vi "MixAndDownsample_5761_stage1.vi"(4 "cosine":fxp<+/-,16,0>, 6 "sine":fxp<+/-,16,0>, 11 "Analog in":i16) -> (0 "data valid":bool, 1 "Q out":fxp<+/-,16,14>, 2 "I out":fxp<+/-,16,14>)   [LabVIEW 2018]
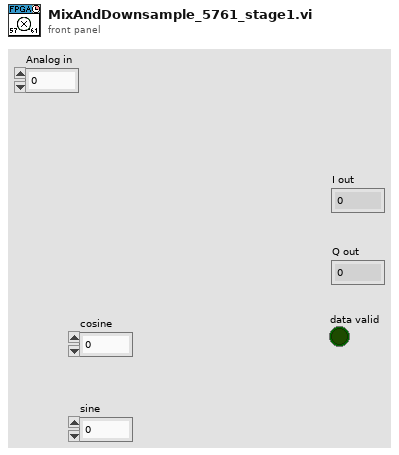
[diagram p1: front panel]
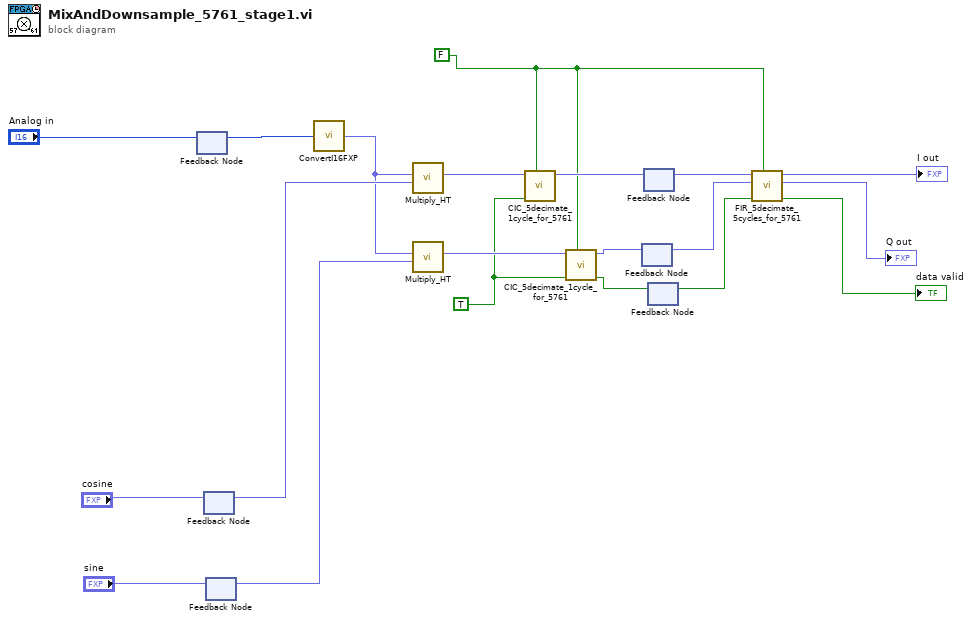
[diagram p0: block diagram]
diagram:
  w4 = FALSE ("reset")
  w11 = TRUE ("valid in")
  n1 = feedback #1() -> (w16:i16)  [unwired: 1 in]
  n2 = feedback-in #1("Analog in") -> ()
  n3 = feedback #2() -> (w17:fxp<+/-,16,0>)  [unwired: 1 in]
  n4 = feedback-in #2("cosine") -> ()
  n5 = feedback #3() -> (w13:fxp<+/-,16,0>)  [unwired: 1 in]
  n6 = feedback-in #3("sine") -> ()
  n7 = call "ConvertI16FXP.vi"("I16"=w16) -> ("y"=w14:fxp<+/-,16,16>)
  n8 = call "Multiply_HT.vi"("DDS sample"=w17, "Signal sample"=w14) -> ("Output"=w15:fxp<+/-,16,14>)  [unwired: 8 in, 1 out]
  n9 = call "Multiply_HT.vi"("DDS sample"=w13, "Signal sample"=w14) -> ("Output"=w12:fxp<+/-,16,14>)  [unwired: 8 in, 1 out]
  n10 = call "CIC_5decimate_1cycle_for_5761.vi"("reset"=w4, "valid in"=w11, "Data in"=w15) -> ("Data out"=w10:fxp<+/-,16,14>)  [unwired: 7 in, 1 out]
  n11 = call "CIC_5decimate_1cycle_for_5761.vi"("reset"=w4, "valid in"=w11, "Data in"=w12) -> ("valid out"=w6:bool, "Data out"=w8:fxp<+/-,16,14>)  [unwired: 7 in]
  n12 = feedback #4() -> (w7:fxp<+/-,16,14>)  [unwired: 1 in]
  n13 = feedback-in #4(w8) -> ()
  n14 = feedback-in #5(w10) -> ()
  n15 = feedback #5() -> (w9:fxp<+/-,16,14>)  [unwired: 1 in]
  n16 = feedback #6() -> (w5:bool)  [unwired: 1 in]
  n17 = feedback-in #6(w6) -> ()
  n18 = call "FIR_5decimate_5cycles_for_5761.vi"("reset"=w4, "valid in"=w5, "Q in"=w7, "I in"=w9) -> ("valid out"=→"data valid":bool, "Q out"=→"Q out":fxp<+/-,16,14>, "I out"=→"I out":fxp<+/-,16,14>)  [unwired: 4 in, 1 out]
